vi "Turn on Display.vi"(6 "chip select (1st chip)":enum16{"1st chip", "2nd chip"}(ring), 8 "error in (no error)":errorcluster, 9 "cursor option":T1(ring)=enum."cursor on & no blink", 10 "display on?":bool=TRUE, 11 "LCD in":u32) -> (0 "error out":errorcluster, 3 "LCD out":u32)   [LabVIEW 2015, in "HD44780 FPGA.lvlib"]
doc: "Turns on/off the display. This VI also sets the status of the cursor after the display is turned on."
uses:
  <vilib>/EmbeddedDisplay/Hitachi HD44780/FPGA/HD44780 FPGA.lvlib
  <vilib>/EmbeddedDisplay/Hitachi HD44780/Common/HD44780 Common.lvlib
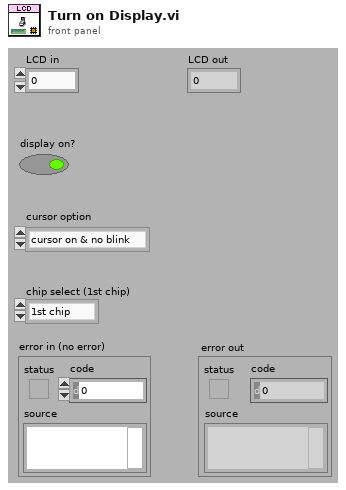
[diagram p1: front panel]
types:
  T1 = enum8{"cursor off", "cursor on & no blink", "cursor on & blink"}
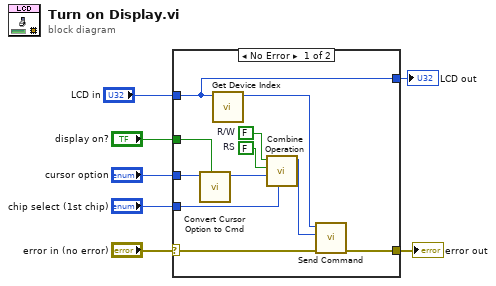
[diagram p0: block diagram]
diagram:
  n1 = case shown="No Error" "error in (no error)" {
    selector: "error in (no error)" -> [w12 w20]
    tunnel: [w11 w20] -> w6
    tunnel: "display on?" -> [w15 _]
    tunnel: "cursor option" -> [w14 _]
    tunnel: "chip select (1st chip)" -> [w13 _]
    tunnel: "LCD in" -> [w8 w19]
    tunnel: [w8 w19] -> w1
    frame No Error {
      w17 = FALSE  # R/W
      w18 = FALSE  # RS
      n2 = call <vilib>:"Convert Cursor Option to Cmd.vi"("display option (on)"=w15, "cursor option"=w14) -> ("Display On Cmd"=w16:u8)  [unwired: 9 in]
      n3 = call <vilib>:"Get Device Index.vi"("LCD in"=w8) -> ("device index"=w9:i8)  [unwired: 10 in]
      n4 = call <vilib>:"Combine Operation.vi"("chip select  (1st chip)"=w13, "cmd/data (0)"=w16, "RS"=w18, "R/W"=w17) -> ("output"=w10:u32)  [unwired: 7 in]
      n5 = call <vilib>:"Send Command.vi"("error in (no error)"=w12, "operation"=w10, "device index"=w9) -> ("error out"=w11:errorcluster)  [unwired: 6 in, 2 out]
    }
    frame Error {
    }
  }
  "error out" <- w6
  "LCD out" <- w1
